vi "UTL_Read_Write Controller 5.vi"(8 "error out":errorcluster) -> (0 "error out 2":errorcluster, 1 "Results C5":dbl[][](array[numeric]), 2 "Recipe":u16, 3 "Running Status":string)   [LabVIEW 2024]
uses:
  <vilib>/Plasmionique/MB Master/MB_Master_Serial/MB_Master_Serial.lvclass
  C:/Program Files (x86)/National Instruments/LabVIEW 2024/vi.lib/Plasmionique/MB Master/MB_Master/MB_Master.lvclass
  Variable global de carga.vi
  <vilib>/Plasmionique/MB Master/MB Master.lvlib
  C:/Program Files (x86)/National Instruments/LabVIEW 2024/vi.lib/Plasmionique/MB Master/MB_Master_Serial/MB_Master_Serial.lvclass
panel:
  in  "Text Ring":u16(ring) items=["Read", "Write"]
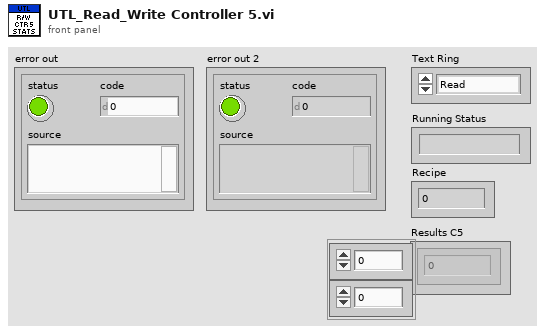
[diagram p1: front panel]
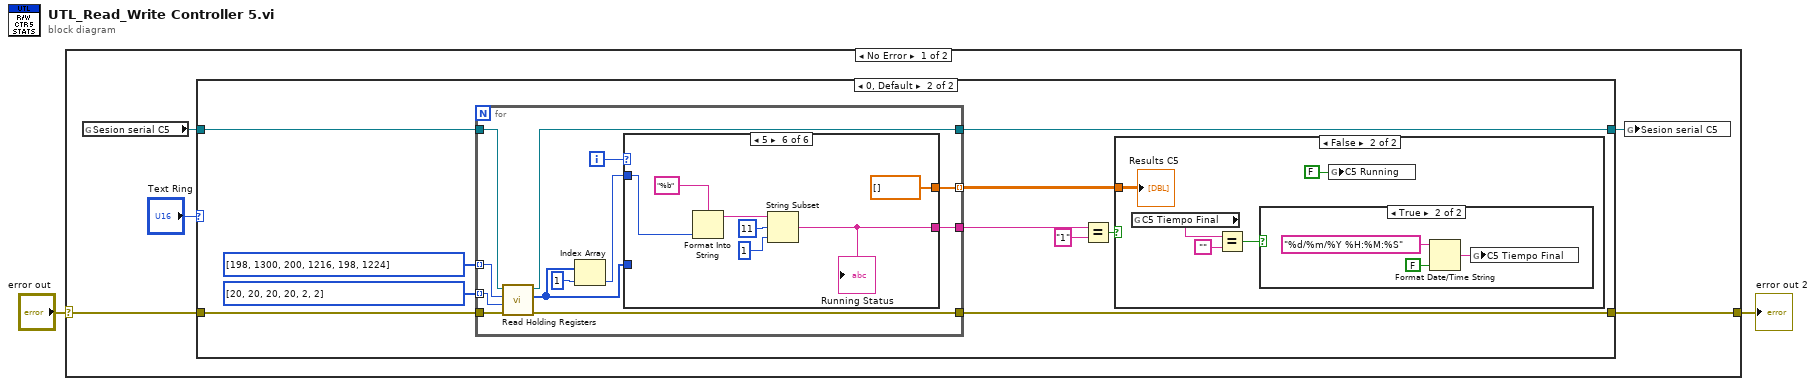
[diagram p0: block diagram]
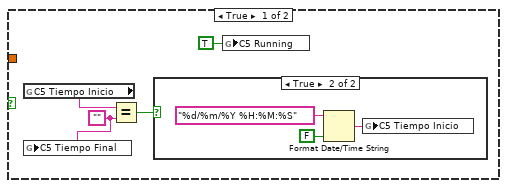
[diagram p3: hidden frame]
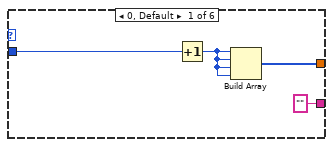
[diagram p6: hidden frame]
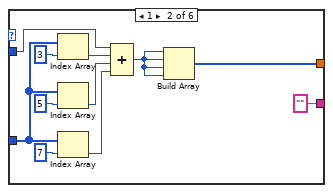
[diagram p7: hidden frame]
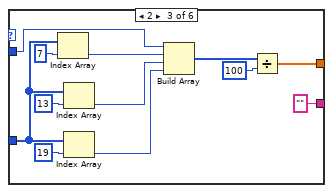
[diagram p8: hidden frame]
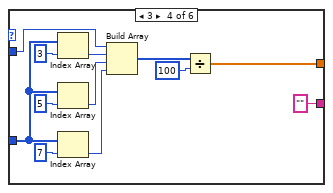
[diagram p9: hidden frame]
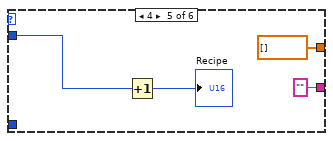
[diagram p10: hidden frame]
diagram:
  n1 = case shown="No Error" "error out" {
    selector: "error out" -> [w6 w97]
    tunnel: [w7 w97] -> w1
    frame No Error {
      n2 = global read "Variable global de carga.vi" "Sesion serial C5"() -> (w4:refnum<class "MB_Master_Serial.lvclass">)
      n3 = case shown="0, Default" "Text Ring" {
        tunnel: [w9 w12] -> w7
        tunnel: w6 -> [w9 w17]
        tunnel: w4 -> [w8 w16]
        tunnel: [w8 w15] -> w3
        frame 1 {
        }
        frame 0, Default {
          n4 = for {
            tunnel: i32[] [198, 1300, 200, 1216, 198, 1224] -> [w42] mode=indexing
            tunnel: [w45] -> w15
            tunnel: [w46] -> w12
            tunnel: [w43] -> w10 mode=indexing
            tunnel: i32[] [20, 20, 20, 20, 2, 2] -> [w41] mode=indexing
            tunnel: w17 -> [w37]
            tunnel: w16 -> [w36]
            tunnel: [w35] -> w14
            i -> [w44]
            n5 = call <vilib>:"Read Holding Registers.vi"("error in (no error)"=w37, "quantity"=w41, "starting address"=w42, "MB session in"=w36) -> ("error out"=w46:errorcluster, "Registers"=w38:u16[], "MB session out"=w45:refnum<class "MB_Master_Serial.lvclass">)  [unwired: 5 in]
            n6 = Index Array(array=w38, index=1) -> (element=w39:u16)
            n7 = case shown="5" w44 {
              tunnel: w38 -> [_ w58 w70 w82 _ _]
              tunnel: [w49 w53 w64 w76 dbl[] [] dbl[] []] -> w43
              tunnel: w39 -> [w48 w52 w63 w75 w89 w92]
              tunnel: ["" "" "" "" "" w90] -> w35
              frame 0, Default {
                n8 = Increment(x=w48) -> (x+1=w50:u16)
                n9 = Build Array(w50, w50, w50, w50) -> (w49:u16[])
              }
              frame 1 {
                n10 = Index Array(array=w58, index=3) -> (element=w57:u16)
                n11 = Index Array(array=w58, index=5) -> (element=w56:u16)
                n12 = Index Array(array=w58, index=7) -> (element=w55:u16)
                n13 = Compound Arithmetic op=ADD(w52, w57, w56, w55) -> (w54:u16)
                n14 = Build Array(w54, w54, w54, w54) -> (w53:u16[])
              }
              frame 2 {
                n15 = Index Array(array=w70, index=7) -> (element=w69:u16)
                n16 = Index Array(array=w70, index=13) -> (element=w68:u16)
                n17 = Index Array(array=w70, index=19) -> (element=w67:u16)
                n18 = Build Array(w63, w69, w68, w67) -> (w65:u16[])
                n19 = Divide(x=w65, y=100) -> (x/y=w64:dbl[])
              }
              frame 3 {
                n20 = Index Array(array=w82, index=3) -> (element=w81:u16)
                n21 = Index Array(array=w82, index=5) -> (element=w80:u16)
                n22 = Index Array(array=w82, index=7) -> (element=w79:u16)
                n23 = Build Array(w75, w81, w80, w79) -> (w78:u16[])
                n24 = Divide(x=w78, y=100) -> (x/y=w76:dbl[])
              }
              frame 4 {
                n25 = Increment(x=w89) -> (x+1=→"Recipe":u16)
              }
              frame 5 {
                n26 = Format Into String(format string="%b", w92) -> (resulting string=w96:string)  [unwired: 2 in, 1 out]
                n27 = String Subset(string=w96, offset (0)=11, length (rest)=1 ("length (rest)")) -> (substring=w90:string)
                "Running Status" <- w90
              }
            }
          }
          n28 = Equal?(x=w14, y="1") -> (x = y?=w11:bool)
          n29 = case shown="False" w11 {
            tunnel: w10 -> [_ w27]
            frame True {
              w20 = ""
              n30 = global read "Variable global de carga.vi" "C5 Tiempo Inicio"() -> (w22:string)
              n31 = global write "Variable global de carga.vi" "C5 Tiempo Final"(w20) -> ()
              n32 = Equal?(x=w22, y=w20) -> (x = y?=w21:bool)
              n33 = case shown="True" w21 {
                frame False {
                }
                frame True {
                  n34 = Format Date/Time String(time format string (%c)="%d/%m/%Y %H:%M:%S", UTC format=FALSE) -> (date/time string=w24:string)  [unwired: 1 in]
                  n35 = global write "Variable global de carga.vi" "C5 Tiempo Inicio"(w24) -> ()
                }
              }
              n36 = global write "Variable global de carga.vi" "C5 Running"(TRUE ("C1 Running")) -> ()
            }
            frame False {
              n37 = global read "Variable global de carga.vi" "C5 Tiempo Final"() -> (w30:string)
              n38 = Equal?(x=w30, y="") -> (x = y?=w29:bool)
              n39 = case shown="True" w29 {
                frame False {
                }
                frame True {
                  n40 = Format Date/Time String(time format string (%c)="%d/%m/%Y %H:%M:%S", UTC format=FALSE) -> (date/time string=w32:string)  [unwired: 1 in]
                  n41 = global write "Variable global de carga.vi" "C5 Tiempo Final"(w32) -> ()
                }
              }
              n42 = global write "Variable global de carga.vi" "C5 Running"(FALSE ("C1 Running")) -> ()
              "Results C5" <- w27
            }
          }
        }
      }
      n43 = global write "Variable global de carga.vi" "Sesion serial C5"(w3) -> ()
    }
    frame Error {
    }
  }
  "error out 2" <- w1
